vi "Matrix Multiple.vi"() -> ()   [LabVIEW 2022 SP3]
uses:
  <vilib>/Analysis/baseanly.llb/A x Vector.vi
  <vilib>/Analysis/NI_AALBase.lvlib
panel:
  out "Output Matrix":dbl[](array[numeric])
  in  "Input Matrix B":dbl[](array[numeric])
  in  "Input Matrix A":dbl[][](array[numeric])
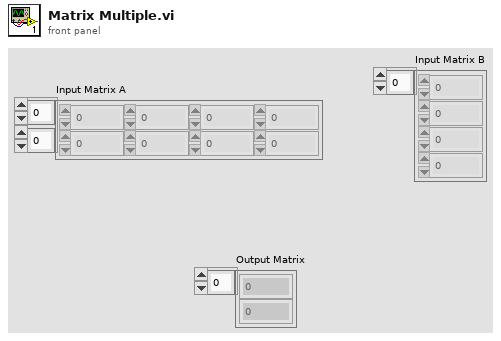
[diagram p1: front panel]
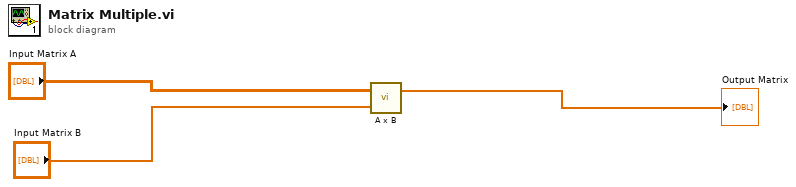
[diagram p0: block diagram]
diagram:
  n1 = call-poly <vilib>:"A x B.vi"("Vector"="Input Matrix B", "A"="Input Matrix A") -> ("A x Vector"=→"Output Matrix":dbl[])  [unwired: 1 out]
